vi "DiffDriveKinematics_Example.vi"() -> ()   [LabVIEW 2019]
uses:
  <vilib>/Rock Robotics/WPI/ThirdParty/JAS_Junk/TrajLib/TypeDef/CHASSIS_SPEEDS.ctl
  <vilib>/Rock Robotics/SystemInterfaces/NetworkCommunication/NetComm_UsageReport_report.vi
  <vilib>/Rock Robotics/WPI/ThirdParty/JAS_Junk/TrajLib/Util_LibraryGlobals.vi
  <vilib>/Rock Robotics/WPI/ThirdParty/JAS_Junk/TrajLib/Trajectory_Library.lvlib
panel:
  out "RightVelocity\nFt/Sec":dbl
  out "LeftVelocity\nFt/Sec":dbl
  out "CHASSIS Speed\nM/S":T1 {"vOmega" format="%10.3f"; "vY" format="%10.3f"; "vX" format="%10.3f"}
  in  "Step":bool
  in  "Right Wheel Velocity\nFt/Sec":dbl
  in  "Left Wheel Velocity\nFT/Sec":dbl
  # "Differential Drive Kinematics Example"
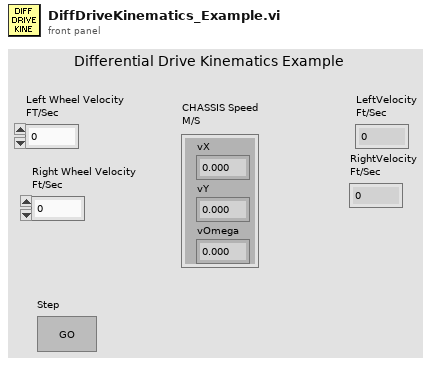
[diagram p1: front panel]
types:
  T1 = typedef "Trajectory_Library.lvlib/CHASSIS_SPEEDS.ctl" = cluster{"vX":dbl, "vY":dbl, "vOmega":dbl}
  T2 = typedef "Trajectory_Library.lvlib/DIFF_DRIVE_KINEMATICS.ctl" = cluster{"TrackWidth_Meters":dbl}
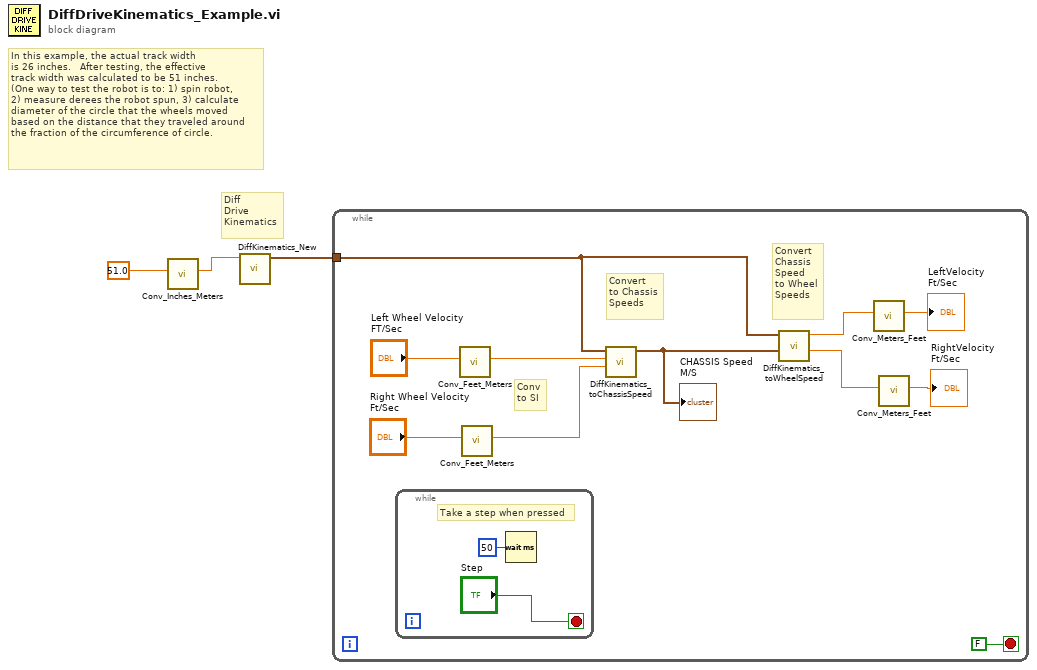
[diagram p0: block diagram]
diagram:
  # "In this example, the actual track width\nis 26 inches.   After testing, the effective\ntrack width was calculated to be 51 inches.\n(One way to test the robot is to: 1) spin robot,\n2) measure derees the robot spun, 3) calculate\ndiameter of the circle that the wheels moved\nbased on the distance that they traveled around\nthe fraction of the circumference of circle."
  # "Diff\nDrive\nKinematics"
  n1 = call <vilib>:"Conv_Inches_Meters.vi"("INCH"=51.0) -> ("Meters"=w3:dbl)  [unwired: 10 in]
  n2 = call <vilib>:"DiffKinematics_New.vi"("TrackWidth_Meters"=w3) -> ("DIFF_DRIVE_KINEMATICS"=w1:T2)  [unwired: 10 in]
  n3 = while {
    tunnel: w1 -> [w10]
    stop <- FALSE stop-if-true
    # "Conv\nto SI"
    # "Convert\nChassis\nSpeed\nto Wheel\nSpeeds"
    # "Convert\nto Chassis\nSpeeds"
    n4 = while {
      stop <- "Step" stop-if-true
      # "Take a step when pressed"
      n5 = Wait (ms)(milliseconds to wait=u32 50) -> ()  [unwired: 1 out]
    }
    n6 = call <vilib>:"Conv_Feet_Meters.vi"("Feet"="Left Wheel Velocity\nFT/Sec") -> ("Meters"=w12:dbl)  [unwired: 10 in]
    n7 = call <vilib>:"Conv_Feet_Meters.vi"("Feet"="Right Wheel Velocity\nFt/Sec") -> ("Meters"=w11:dbl)  [unwired: 10 in]
    n8 = call <vilib>:"DiffKinematics_toChassisSpeed.vi"("RightVelocity"=w11, "LeftVelocity"=w12, "inDIFF_DRIVE_KINEMATICS"=w10) -> ("CHASSIS Speed"=w9:T1)  [unwired: 8 in]
    "CHASSIS Speed\nM/S" <- w9
    n9 = call <vilib>:"DiffKinematics_toWheelSpeed.vi"("CHASSIS Speed"=w9, "DIFF_DRIVE_KINEMATICS"=w10) -> ("RightVelocity"=w4:dbl, "LeftVelocity"=w5:dbl)  [unwired: 8 in]
    n10 = call <vilib>:"Conv_Meters_Feet.vi"("Meters"=w5) -> ("Feet"=→"LeftVelocity\nFt/Sec":dbl)  [unwired: 10 in]
    n11 = call <vilib>:"Conv_Meters_Feet.vi"("Meters"=w4) -> ("Feet"=→"RightVelocity\nFt/Sec":dbl)  [unwired: 10 in]
  }
